vi "Create Command Array Channel_Type Cast.vi"(8 "Error In":errorcluster, 10 "Settings":T1, 11 "Message Refnum In":T4=18446744073709551615 format="%.0x") -> (0 "Error Out":errorcluster, 2 "Channel Refnums":T4[](array[typedef]) format="%.0x", 3 "Message Refnum Out":T4=18446744073709551615 format="%.0x")   [LabVIEW 2020, in "Scripting API.lvlib"]
uses:
  Scripting API.lvlib
  <vilib>/NI VeriStand/Custom Device API/Custom Device Item Ref.ctl
  Examples/Control 11.ctl
  Examples/Control 13.ctl
  Examples/Control 12.ctl
  <vilib>/NI VeriStand/Custom Device API/Custom Device API.lvlib
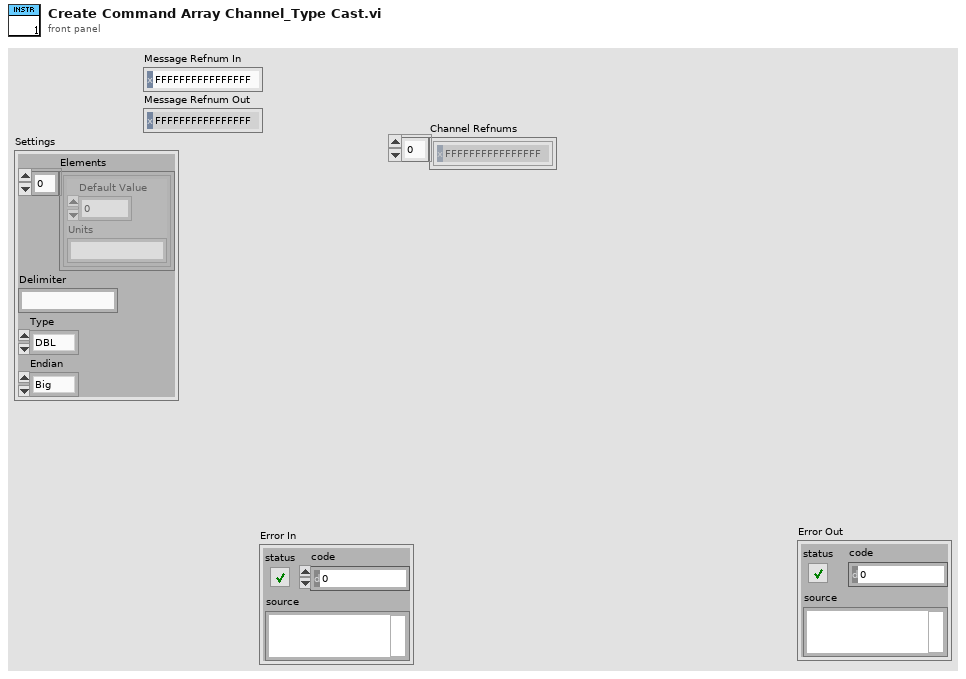
[diagram p1: front panel]
types:
  T1 = typedef "Control 11.ctl" = cluster{"Elements":cluster{"Default Value":dbl, "Units":string}[], "Delimiter":string, "Type":T2, "Endian":T3}
  T2 = typedef "Control 13.ctl" = enum16{"DBL"}
  T3 = typedef "Control 12.ctl" = enum16{"Big", "Little", "Native"}
  T4 = typedef "Custom Device API.lvlib/Custom Device Item Ref.ctl" = u64
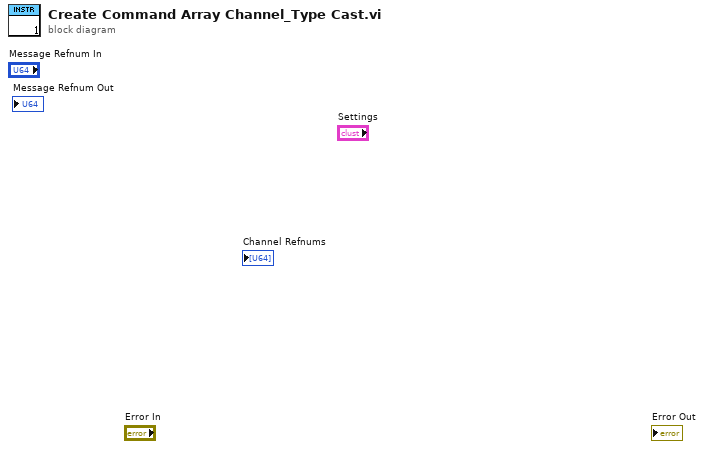
[diagram p0: block diagram]
diagram:
